vi "Connect Trigger Terminals.vi"(8 "error in (no error)":errorcluster, 10 "Routing Information":T1={"Source"="PXI_Trig0", "Destination"="PXI_Trig0", "Synchronization Clock"="SyncClkAsync"}, 11 "instrument handle":refnum<k15>) -> (0 "error out":errorcluster, 3 "instrument handle out":refnum<k15>)   [LabVIEW 2026]
doc: "This VI allows an array input of Trigger Routing Controls. NI-SYNC will make the connects of each array input. The benefit of this vi is there is no need for multiple string inputs."
uses:
  Trigger Routing.ctl
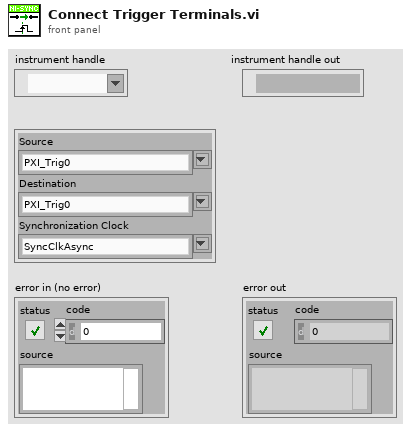
[diagram p1: front panel]
types:
  T1 = typedef "Trigger Routing.ctl" = cluster{"Source":string, "Destination":string, "Synchronization Clock":string}
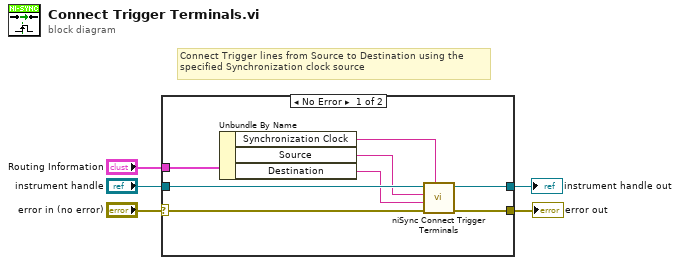
[diagram p0: block diagram]
diagram:
  # "Connect Trigger lines from Source to Destination using the\nspecified Synchronization clock source"
  n1 = case shown="No Error" "error in (no error)" {
    selector: "error in (no error)" -> [w10 w15]
    tunnel: "Routing Information" -> [w13 _]
    tunnel: "instrument handle" -> [w12 w14]
    tunnel: [w11 w14] -> w4
    tunnel: [w9 w15] -> w2
    frame No Error {
      n2 = Unbundle By Name(w13) -> ("Synchronization Clock"=w8:string, "Source"=w7:string, "Destination"=w6:string)
      n3 = call <instrlib>:"niSync Connect Trigger Terminals.vi"("synchronization clock"=w8, "error in (no error)"=w10, "destination terminal"=w6, "source terminal"=w7, "instrument handle"=w12) -> ("error out"=w9:errorcluster, "instrument handle out"=w11:refnum<k15>)  [unwired: 5 in]
    }
    frame Error {
    }
  }
  "instrument handle out" <- w4
  "error out" <- w2
